vi "Current Encoder Values.vi"   [LabVIEW 2019]
uses:
  <vilib>/Rock Robotics/WPI/Utilities/WPI_GetSetVariantRefNum.vi
  <vilib>/Rock Robotics/WPI/ThirdParty/Phoenix-LabVIEW/Motor Controller/Get/CTRE_Phoenix_MotorController_GetSelectedSensorData.vi
  Robot Global Data.vi
types:
  T1 = typedef "WPI_RobotDriveDevRef.ctl" = cluster{"DevStatus":errorcluster, "Motors[]":T2[], "Square Inputs":bool, "Max Output":dbl}
  T2 = typedef "WPI_MotorControlDeviceRef.ctl" = cluster{"DeviceStatus":errorcluster, "Type":T3, "PWM":cluster{"PWM Channel":T4, "DeadBand":T5}, "CAN":cluster{"Device Number":u8, "SetOutput VI Ref":variant, "GetOutput VI Ref":variant, "Enable VI Ref":variant, "Disable VI Ref":variant, "Data":variant}, "Invert":bool, "DIO PWM":cluster{"PWM \"Enable\" Channel":T4, "DIOChannel":T6, "PWM Rate":dbl}}
  T3 = typedef "WPI_MotorControlType.ctl" = enum16{"PWM", "CAN", "DIO PWM"}
  T4 = typedef "FPGA_DIOPWMChannel.ctl" = enum8{"PWM 0", "PWM 1", "PWM 2", "PWM 3", "PWM 4", "PWM 5", "PWM 6", "PWM 7", "PWM 8", "PWM 9", "PWM MXP 0", "PWM MXP 1", "PWM MXP 2", "PWM MXP 3", "PWM MXP 4", "PWM MXP 5", "PWM MXP 6", "PWM MXP 7", "PWM MXP 8", "PWM MXP 9", "Invalid"}
  T5 = typedef "WPI_PWMDeadband.ctl" = cluster{"Name":string, "maxPositivePwm":i32, "minPositivePwm":i32, "centerPwm":i32, "maxNegativePwm":i32, "minNegativePwm":i32, "angularRange":u16}
  T6 = typedef "FPGA_DIOChannel.ctl" = enum8{"DIO 0", "DIO 1", "DIO 2", "DIO 3", "DIO 4", "DIO 5", "DIO 6", "DIO 7", "DIO 8", "DIO 9", "DIO MXP 0", "DIO MXP 1", "DIO MXP 2", "DIO MXP 3", "DIO MXP 4", "DIO MXP 5", "DIO MXP 6", "DIO MXP 7", "DIO MXP 8", "DIO MXP 9", "DIO MXP 10", "DIO MXP 11", "DIO MXP 12", "DIO MXP 13", "DIO MXP 14", "DIO MXP 15", "SPI Port CS1", "SPI Port CS2", "SPI Port CS3", "SPI Port MISO", "SPI Port MOSI", "Invalid"}
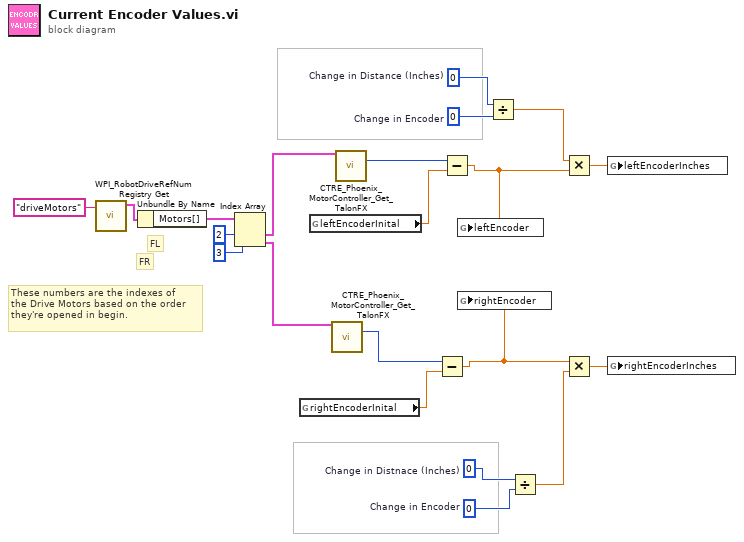
[diagram p0: block diagram]
diagram:
  w13 = 0  # Change in Encoder
  w12 = 0  # Change in Distnace (Inches)
  w16 = 0  # Change in Encoder
  w15 = 0  # Change in Distance (Inches)
  # "FR"
  # "FL"
  # "These numbers are the indexes of \nthe Drive Motors based on the order\nthey're opened in begin."
  n1 = call <vilib>:"WPI_RobotDriveRefNum Registry Get.vi"("refnum name"="driveMotors") -> ("RobotDriveDevRef"=w2:T1)  [unwired: 9 in, 1 out]
  n2 = Unbundle By Name(w2) -> ("Motors[]"=w3:T2[])
  n3 = Index Array(array=w3, index #1=2 ("index"), index #2=3 ("index")) -> (element #1=w6:T2, element #2=w7:T2)
  n4 = global read "Robot Global Data.vi" "rightEncoderInital"() -> (w11:dbl)
  n5 = global read "Robot Global Data.vi" "leftEncoderInital"() -> (w9:dbl)
  n6 = call-poly <vilib>:"CTRE_Phoenix_MotorController_Get_TalonFX.vi"("PhoenixMotorControlDevRef"=w7) -> ("Position (Raw Sensor Units)"=w10:i32)  [unwired: 11 in, 3 out]
  n7 = call-poly <vilib>:"CTRE_Phoenix_MotorController_Get_TalonFX.vi"("PhoenixMotorControlDevRef"=w6) -> ("Position (Raw Sensor Units)"=w8:i32)  [unwired: 11 in, 3 out]
  n8 = Subtract(x=w10, y=w11) -> (x-y=w18:dbl)
  n9 = Subtract(x=w8, y=w9) -> (x-y=w19:dbl)
  n10 = global write "Robot Global Data.vi" "leftEncoder"(w19) -> ()
  n11 = global write "Robot Global Data.vi" "rightEncoder"(w18) -> ()
  n12 = Divide(x=w15, y=w16) -> (x/y=w17:dbl)
  n13 = Divide(x=w12, y=w13) -> (x/y=w14:dbl)
  n14 = Multiply(x=w17, y=w19) -> (x*y=w20:dbl)
  n15 = Multiply(x=w18, y=w14) -> (x*y=w21:dbl)
  n16 = global write "Robot Global Data.vi" "leftEncoderInches"(w20) -> ()
  n17 = global write "Robot Global Data.vi" "rightEncoderInches"(w21) -> ()
